vi "Magazine_Globals.vi"() -> ()   [LabVIEW 2019]
uses:
  Subsystems/Magazine/Magazine_Cluster.ctl
  Subsystems/Magazine/Magazine_States.ctl
  Utility VIs/Basic_Motor_Modes.ctl
panel:
  in  "Manual_Magazine_Power":dbl
  in  "Magazine_Firing_Throttle":dbl
  in  "Magazine_Motor_Mode":T1
  in  "Magazine_Horizontal_Throttle":dbl
  in  "Magazine_Vertical_Throttle":dbl
  in  "Magazine_Execute_Notifier":refnum<notifier>
  in  "Magazine_Set_Notifier":refnum<notifier>
  in  "Magazine_Execute_Ref":string="Magazine_Execute_Ref"
  in  "Magazine_Set_Ref":string="Magazine_Set_Ref"
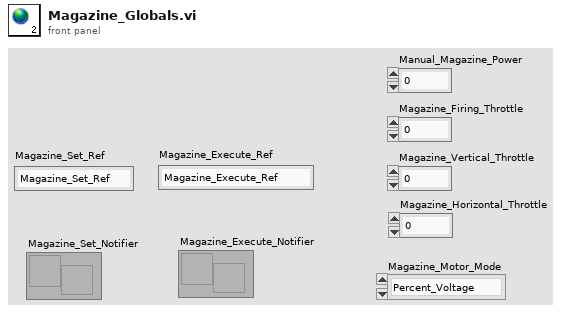
[diagram p1: front panel]
types:
  T1 = typedef "Basic_Motor_Modes.ctl" = enum16{"Percent_Voltage", "Speed_Control", "Position_Control", "Current"}
diagram:
